vi "GetPaneRefFromPosition.vi"(8 "error in (no error)":errorcluster, 10 "Position":T1 items=["Top", "Left", "Center", "Right", "Bottom"], 11 "PentaPanesGUI in":refnum<class "PentaPanes.lvclass">) -> (0 "error out":errorcluster, 2 "PaneRef":refnum<vi>, 3 "PentaPanesGUI out":refnum<class "PentaPanes.lvclass">)   [LabVIEW 2022 SP3, in "PentaPanesLibrary.lvlib" / "PentaPanes.lvclass"]
doc: "This VI reads the Pane's position string and Label.\n\nPaneRef - A reference to the pane. \nPos String - Outputs a position string (\"Top\", \"Left\", \"Right\", \"Bottom\").\nLabel.Text - Outputs The Label of the pane."
uses:
  PentaPanes.lvclass
  PanePosition.ctl
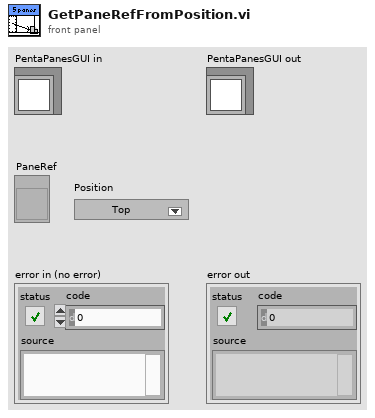
[diagram p1: front panel]
types:
  T1 = typedef "PentaPanesLibrary.lvlib/PentaPanes.lvclass/PanePosition.ctl" = u16
  T2 = typedef "PentaPanesLibrary.lvlib/PentaPanes.lvclass/PanesCluster.ctl" = cluster{"Top Pane":refnum<vi>, "Left Pane":refnum<vi>, "Center Pane":refnum<vi>, "Right Pane":refnum<vi>, "Bottom Pane":refnum<vi>}
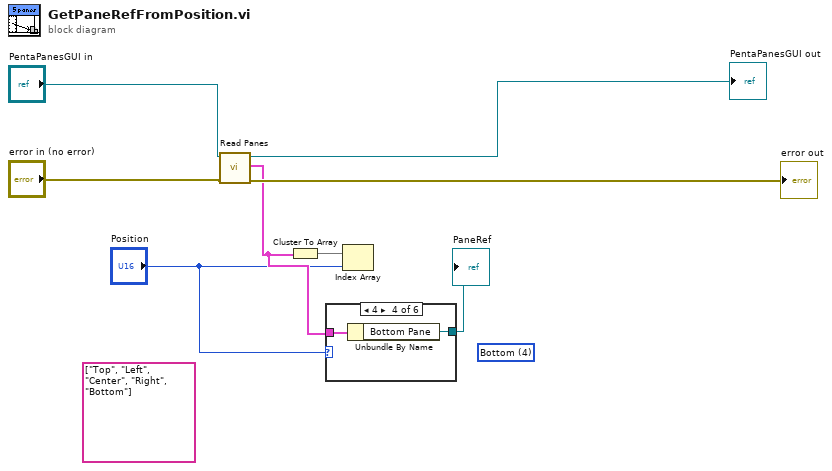
[diagram p0: block diagram]
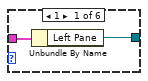
[diagram p2: hidden frame]
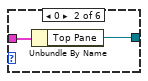
[diagram p3: hidden frame]
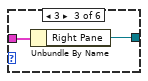
[diagram p4: hidden frame]
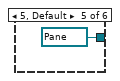
[diagram p5: hidden frame]
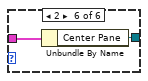
[diagram p6: hidden frame]
diagram:
  (unwired) u16 4 items=["Top", "Left", "Center", "Right", "Bottom"] ("Position")
  (unwired) string[] ["Top", "Left", "Center", "Right", "Bottom"]
  n1 = call-dynamic "Read Panes.vi"("error in (no error)"="error in (no error)", "PentaPanesGUI in"="PentaPanesGUI in") -> ("error out"=→"error out":errorcluster, "Panes"=w3:T2, "PentaPanesGUI out"=→"PentaPanesGUI out":refnum<class "PentaPanes.lvclass">)  [unwired: 7 in]
  n2 = Cluster To Array(cluster=w3) -> (array=w4:refnum<vi>[])
  n3 = case shown="4" "Position" {
    tunnel: w3 -> [w10 w12 w14 w16 _ w19]
    tunnel: [w9 w11 w13 w15 refnum<vi> refnum ("Center Pane") w18] -> w1
    frame 1 {
      n4 = Unbundle By Name(w10) -> ("Left Pane"=w9:refnum<vi>)
    }
    frame 0 {
      n5 = Unbundle By Name(w12) -> ("Top Pane"=w11:refnum<vi>)
    }
    frame 3 {
      n6 = Unbundle By Name(w14) -> ("Right Pane"=w13:refnum<vi>)
    }
    frame 4 {
      n7 = Unbundle By Name(w16) -> ("Bottom Pane"=w15:refnum<vi>)
    }
    frame 5, Default {
    }
    frame 2 {
      n8 = Unbundle By Name(w19) -> ("Center Pane"=w18:refnum<vi>)
    }
  }
  "PaneRef" <- w1
  n9 = Index Array(array=w4, index="Position") -> ()  [unwired: 1 out]
